vi "Read Time.vi"(8 "error in (no error)":errorcluster, 11 "PanelCloseMsg in":refnum<class "PanelCloseMsg.lvclass">) -> (0 "error out":errorcluster, 2 "Time":u32, 3 "PanelCloseMsg out":refnum<class "PanelCloseMsg.lvclass">)   [LabVIEW 2020, in "ActorEvents.lvlib" / "PanelCloseMsg.lvclass"]
uses:
  <vilib>/gpm_packages/@cs/mva-viewable/Source/ActorEvents/IEventAggregator Messages/PanelCloseMsg/PanelCloseMsg.lvclass
  <vilib>/gpm_packages/@cs/mva-viewable/Source/ActorEvents/IEventAggregator Messages/PanelCloseMsg/PanelCloseMsg.lvclass/PanelCloseMsg.ctl
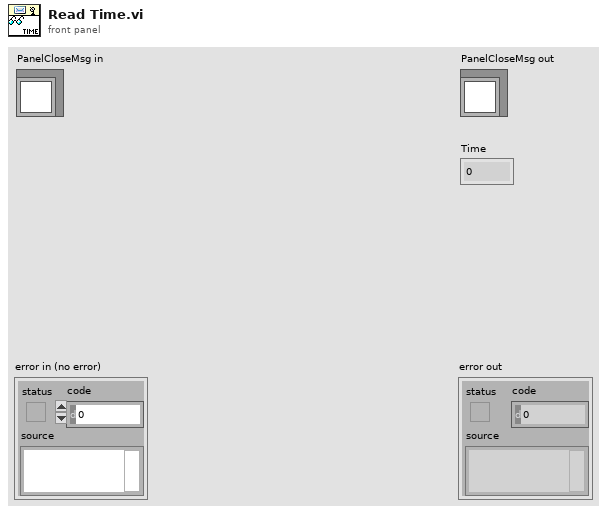
[diagram p1: front panel]
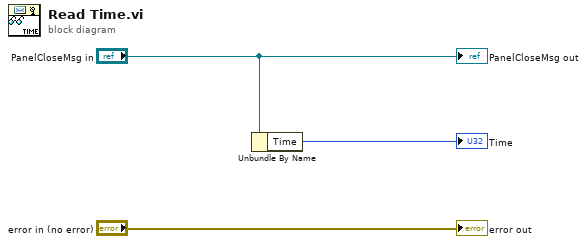
[diagram p0: block diagram]
diagram:
  n1 = Unbundle By Name("PanelCloseMsg in") -> ("Time"=→"Time":u32)
  "error out" <- "error in (no error)"
  "PanelCloseMsg out" <- "PanelCloseMsg in"
